vi "GetData.vi"() -> (3 "Array":T1(array[cluster]))   [LabVIEW 2017]
uses:
  <vilib>/Utility/config.llb/Read Key (String).vi
  <vilib>/Utility/config.llb/NI_LVConfig.lvlib
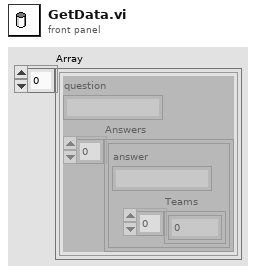
[diagram p1: front panel]
types:
  T1 = cluster{"question":string, "Answers":cluster{"answer":string, "Teams":i32[]}[]}[]
  T2 = typedef "NI_LVConfig.lvlib/Config Data RefNum.ctl" = refnum<k1>
  T3 = cluster{"question":string, "Answers":cluster{"answer":string, "Teams":i32[]}[]}
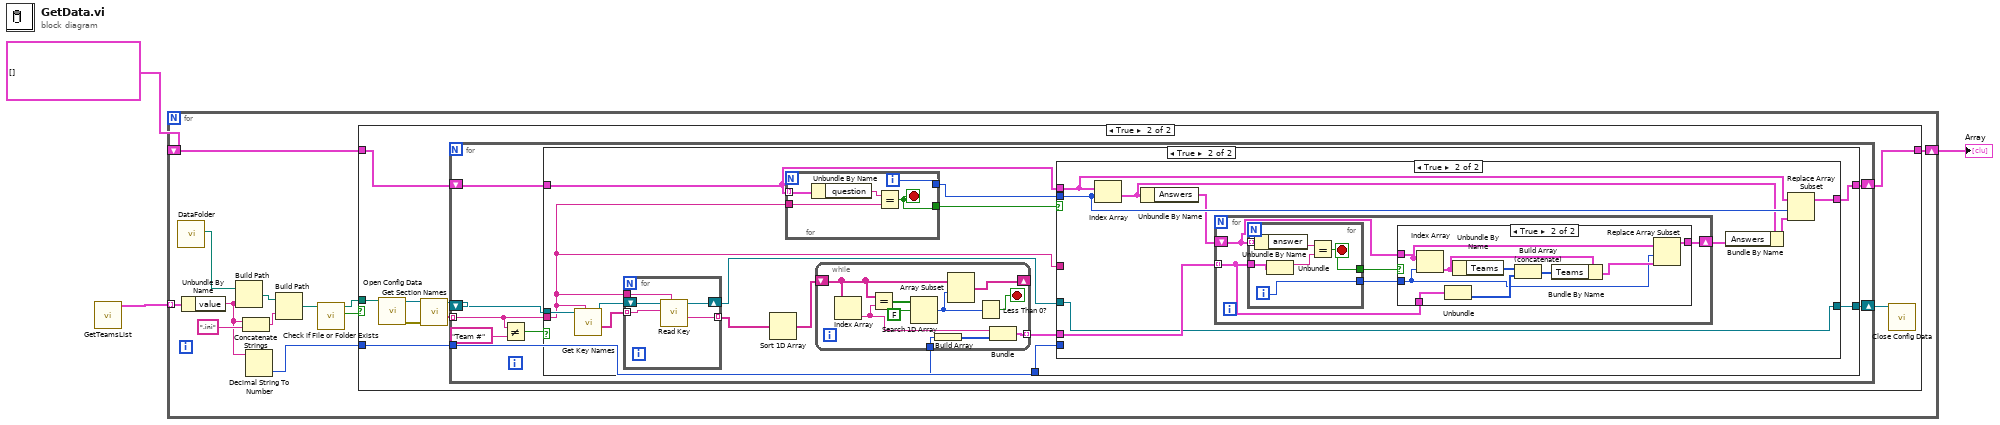
[diagram p0: block diagram]
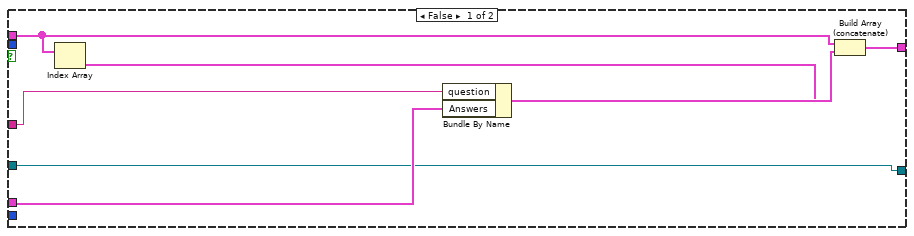
[diagram p4: hidden frame]
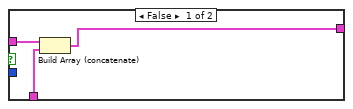
[diagram p5: hidden frame]
diagram:
  n1 = call "GetTeamsList.vi"() -> ("Array"=w1:cluster{string, "value":string}[])  [unwired: 11 in]
  n2 = for {
    tunnel: w1 -> [w15] mode=indexing
    shift-right: [w7] -> w3
    shift-left: T1 [] -> [w8]
    n3 = call "DataFolder.vi"() -> ("appended path"=w14:path)  [unwired: 11 in]
    n4 = Unbundle By Name(w15) -> ("value"=w5:string)
    n5 = Build Path(base path=w14, name or relative path=w5) -> (appended path=w13:path)
    n6 = Concatenate Strings(w5, ".ini" ("string")) -> (w12:string)
    n7 = Decimal String To Number(string=w5) -> (number=w4:i32)  [unwired: 2 in, 1 out]
    n8 = Build Path(base path=w13, name or relative path=w12) -> (appended path=w10:path)
    n9 = call <vilib>:"Check if File or Folder Exists.vi"("path"=w10) -> ("file or folder exists?"=w9:bool, "dup path"=w6:path)  [unwired: 8 in, 1 out]
    n10 = case shown="True" w9 {
      tunnel: w8 -> [w16 w20]
      tunnel: [w16 w19] -> w7
      tunnel: w6 -> [_ w25]
      tunnel: w4 -> [_ w18]
      frame False {
      }
      frame True {
        n11 = call <vilib>:"Open Config Data.vi"("configuration file path"=w25) -> ("error out"=w24:errorcluster, "refnum"=w23:T2)  [unwired: 8 in, 1 out]
        n12 = call <vilib>:"Get Section Names.vi"("error in (no error)"=w24, "refnum"=w23) -> ("section names"=w22:string[], "refnum out"=w21:T2)  [unwired: 7 in, 1 out]
        n13 = for {
          tunnel: w22 -> [w28] mode=indexing
          shift-right: [w32] -> w19
          shift-left: w20 -> [w31]
          tunnel: w18 -> [w29]
          shift-right: [w30] -> w17
          shift-left: w21 -> [w33]
          n14 = Not Equal?(x=w28, y="Team #") -> (x != y?=w26:bool)
          n15 = case shown="True" w26 {
            tunnel: w33 -> [w35 w48]
            tunnel: [w34 w47] -> w32
            tunnel: w31 -> [w34 w46]
            tunnel: [w35 w38] -> w30
            tunnel: w29 -> [_ w37]
            tunnel: w28 -> [_ w36]
            frame False {
            }
            frame True {
              n16 = call <vilib>:"Get Key Names.vi"("section"=w36, "refnum"=w48) -> ("key names"=w42:string[], "refnum out"=w41:T2)  [unwired: 6 in, 2 out]
              n17 = for {
                tunnel: w42 -> [w54] mode=indexing
                shift-right: [w52] -> w39
                shift-left: w41 -> [w53]
                tunnel: w36 -> [w51]
                tunnel: [w50] -> w40 mode=indexing
                n18 = call-poly <vilib>:"Read Key.vi"("section"=w51, "key"=w54, "refnum"=w53) -> ("value"=w50:string, "refnum out"=w52:T2)  [unwired: 5 in, 2 out]
              }
              n19 = Sort 1D Array(array=w40) -> (sorted array=w44:string[])
              n20 = for {
                tunnel: w46 -> [w108] mode=indexing
                tunnel: w36 -> [w106]
                tunnel: [w105] -> w45
                tunnel: [w104] -> w49
                i -> [w105]
                stop <- w104 stop-if-true
                n21 = Unbundle By Name(w108) -> ("question"=w107:string)
                n22 = Equal?(x=w107, y=w106) -> (x = y?=w104:bool)
              }
              n23 = while {
                tunnel: w37 -> [w64]
                tunnel: [w63] -> w43 mode=indexing
                shift-right: [w57] -> _
                shift-left: w44 -> [w60]
                stop <- w55 stop-if-true
                n24 = Index Array(array=w60) -> (element=w59:string)  [unwired: 1 in]
                n25 = Equal?(x=w60, y=w59) -> (x = y?=w62:bool[])
                n26 = Search 1D Array(1D array=w62, element=FALSE) -> (index of element=w56:i32)  [unwired: 1 in]
                n27 = Build Array(w64) -> (w58:i32[])
                n28 = Array Subset(array=w60, index=w56) -> (w57:string[])  [unwired: 1 in]
                n29 = Less Than 0?(x=w56) -> (x < 0?=w55:bool)
                n30 = Bundle("value"=w59, w58) -> (w63:cluster{"value":string, i32[]})  [unwired: 1 in]
              }
              n31 = case shown="True" w49 {
                tunnel: w46 -> [w71 w79]
                tunnel: w39 -> [w65 w75]
                tunnel: w36 -> [w70 _]
                tunnel: [w68 w80] -> w47
                tunnel: w37 -> [_ _]
                tunnel: w45 -> [_ w78]
                tunnel: w43 -> [w66 w76]
                tunnel: [w65 w75] -> w38
                frame False {
                  n32 = Index Array(array=w71) -> (element=w67:T3)  [unwired: 1 in]
                  n33 = Bundle By Name(cluster=w67, "question"=w70, "Answers"=w66) -> (w69:T3)
                  n34 = Build Array (concatenate)(w71, w69) -> (w68:T1)
                }
                frame True {
                  n35 = Index Array(array=w79, index=w78) -> (element=w72:T3)
                  n36 = Unbundle By Name(w72) -> ("Answers"=w77:cluster{"answer":string, "Teams":i32[]}[])
                  n37 = for {
                    tunnel: w76 -> [w82] mode=indexing
                    shift-right: [w83] -> w74
                    shift-left: w77 -> [w84]
                    n38 = for {
                      tunnel: w84 -> [w103] mode=indexing
                      tunnel: w82 -> [w102]
                      tunnel: [w99] -> w85
                      tunnel: [w98] -> w81
                      i -> [w98]
                      stop <- w99 stop-if-true
                      n39 = Unbundle By Name(w103) -> ("answer"=w101:string)
                      n40 = Unbundle(w102) -> ("value"=w100:string)  [unwired: 1 out]
                      n41 = Equal?(x=w101, y=w100) -> (x = y?=w99:bool)
                    }
                    n42 = case shown="True" w85 {
                      tunnel: w84 -> [w88 w91]
                      tunnel: [w87 w89] -> w83
                      tunnel: w82 -> [w86 w96]
                      tunnel: w81 -> [_ w90]
                      frame False {
                        n43 = Build Array (concatenate)(w88, w86) -> (w87:cluster{"value":string, "Teams":i32[]}[])
                      }
                      frame True {
                        n44 = Index Array(array=w91, index=w90) -> (element=w94:cluster{"answer":string, "Teams":i32[]})
                        n45 = Unbundle(w96) -> (w95:i32[])  [unwired: 1 out]
                        n46 = Unbundle By Name(w94) -> ("Teams"=w97:i32[])
                        n47 = Build Array (concatenate)(w97, w95) -> (w93:i32[])
                        n48 = Bundle By Name(cluster=w94, "Teams"=w93) -> (w92:cluster{"answer":string, "Teams":i32[]})
                        n49 = Replace Array Subset(array=w91, new element=w92, index=w90) -> (w89:cluster{"answer":string, "Teams":i32[]}[])
                      }
                    }
                  }
                  n50 = Bundle By Name(cluster=w72, "Answers"=w74) -> (w73:T3)
                  n51 = Replace Array Subset(array=w79, new element=w73, index=w78) -> (w80:T1)
                }
              }
            }
          }
        }
        n52 = call <vilib>:"Close Config Data.vi"("refnum"=w17) -> ()  [unwired: 9 in, 2 out]
      }
    }
  }
  "Array" <- w3
